vi "Configure Amplitude Sweep at Constant Frequency.vi"(0 "template configuration":refnum<class "SV Signal.lvclass">, 1 "frequency (Hz)":dbl=1000.0, 5 "amplitude range":cluster{"start":dbl, "stop":dbl}={"start"=10.0, "stop"=10000.0} {"stop" format="%.2f"; "start" format="%.2f"}, 7 "number of steps":i32=100 min=1, 9 "profile":enum16{"Linear", "Logarithmic"}(ring)=enum."Logarithmic", 11 "error in (no error)":errorcluster) -> (4 "signal configuration":refnum<class "SV Discrete Sweep.lvclass">, 15 "error out":errorcluster)   [LabVIEW 2017, in "SV Discrete Sweep.lvclass"]
doc: "Configures a user-defined test signal. Wire the outputs to SV Signal (waveform) VI to generate the test signal, or wire to SV Signal Property Node to configure additional parameters before wiring to the SV Signal (waveform) VI."
uses:
  <vilib>/addons/_NISVFA/_Generation/Signal Generation/SV Discrete Sweep/SV Discrete Sweep.lvclass
  C:/Program Files (x86)/National Instruments/LabVIEW 2017/vi.lib/addons/_NISVFA/_Generation/Signal Generation/SV Signal/SV Signal.lvclass
  C:/Program Files (x86)/National Instruments/LabVIEW 2017/vi.lib/addons/_NISVFA/_Generation/Signal Generation/SV Function/SV Function.lvclass
  <vilib>/addons/_NISVFA/_Generation/Signal Generation/SV Signal/SV Signal.lvclass
  <vilib>/addons/_NISVFA/_Generation/Signal Generation/SV Signal/sv_System Timing Model.ctl
  <vilib>/addons/_NISVFA/_Generation/Signal Generation/SV Discrete Sweep/SV Discrete Sweep.lvclass/SV Discrete Sweep.ctl
  <vilib>/addons/_NISVFA/_Generation/Signal Generation/SV Signal/Write Sample Rate.vi
  <vilib>/addons/_NISVFA/_Generation/Signal Generation/SV Signal/Write System Timing Model.vi
  <vilib>/addons/_NISVFA/_Generation/Signal Generation/SV Function/Write Measurement Cycles.vi
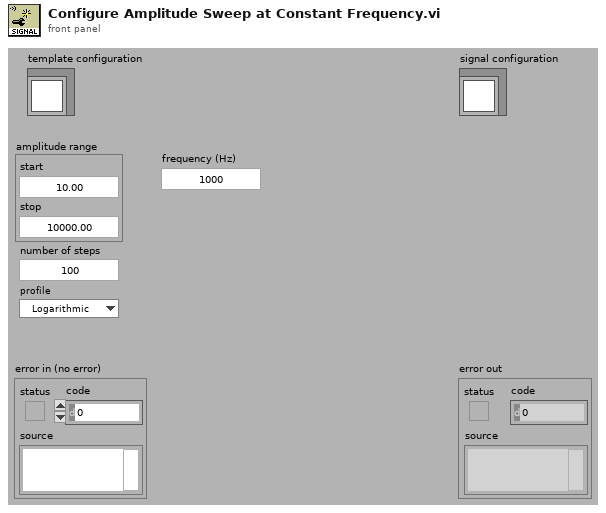
[diagram p1: front panel]
types:
  T1 = cluster{"start":dbl, "stop":dbl, "number of steps":i32}
  T2 = typedef "SV Signal.lvclass/sv_System Timing Model.ctl" = i64
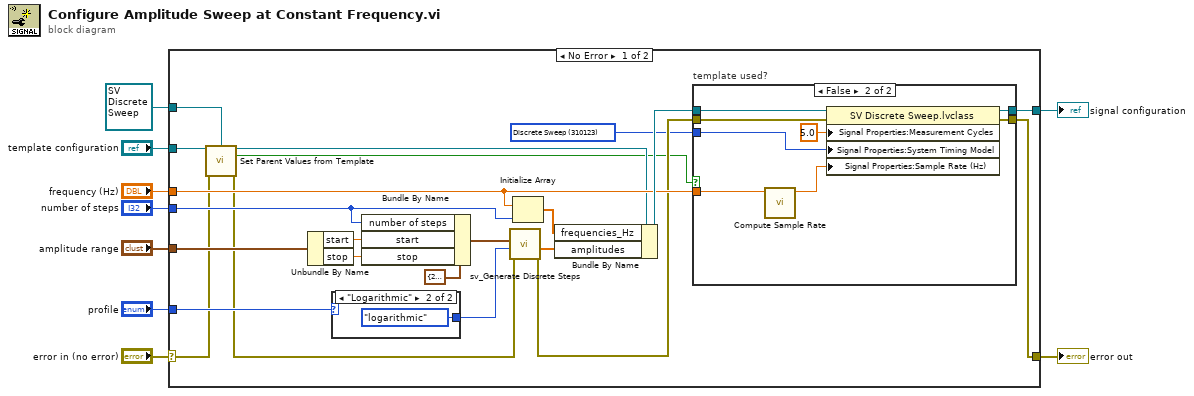
[diagram p0: block diagram]
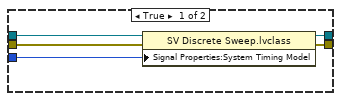
[diagram p2: hidden frame]
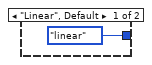
[diagram p3: hidden frame]
diagram:
  n1 = case shown="No Error" "error in (no error)" {
    selector: "error in (no error)" -> [w13 w47]
    tunnel: [w20 w47] -> w8
    tunnel: [w22 w48] -> w6
    tunnel: refnum<class "SV Discrete Sweep.lvclass"> refnum ("Discrete Frequency Sweep") -> [w14 w48]
    tunnel: "amplitude range" -> [w31 _]
    tunnel: "number of steps" -> [w18 _]
    tunnel: "profile" -> [w26 _]
    tunnel: "frequency (Hz)" -> [w19 _]
    tunnel: "template configuration" -> [w16 _]
    frame No Error {
      w10 = T2 310123 items=["Finite"=10178, "-"=-1, "Continuous"=10123, "-"=-2, "Settled"=110123, "Averaged"=210123, "Discrete Sweep"=310123, "Continuous Sweep"=410123] ("System Timing Model")
      n2 = call-dynamic "Set Parent Values from Template.vi"("template configuration"=w16, "signal configuration in"=w14, "error in (no error)"=w13) -> ("signal configuration out"=w15:refnum<class "SV Discrete Sweep.lvclass">, "template used?"=w11:bool, "error out"=w12:errorcluster)  [unwired: 10 in]
      n3 = Unbundle By Name(w31) -> ("start"=w29:dbl, "stop"=w28:dbl)
      n4 = case shown="\"Logarithmic\"" w26 {
        tunnel: [enum16{"linear", "logarithmic"}."linear" ("frequency spacing") enum16{"linear", "logarithmic"}."logarithmic" ("frequency spacing")] -> w25
        frame "Linear", Default {
        }
        frame "Logarithmic" {
        }
      }
      n5 = Bundle By Name(cluster=T1 {"start"=20.0, "stop"=20000.0, "number of steps"=100} ("sweep frequencies"), "number of steps"=w18, "start"=w29, "stop"=w28) -> (w27:T1)
      n6 = call <vilib>:"sv_Generate Discrete Steps.vi"("error in (no error)"=w12, "spacing"=w25, "steps"=w27) -> ("error out"=w17:errorcluster, "frequency list"=w24:dbl[])  [unwired: 7 in]
      n7 = Initialize Array(w19, w18) -> (w21:dbl[])
      n8 = Bundle By Name(cluster=w15, "frequencies_Hz"=w21, "amplitudes"=w24) -> (w23:refnum<class "SV Discrete Sweep.lvclass">)
      n9 = case "template used?" shown="False" w11 {
        tunnel: w23 -> [w36 w44]
        tunnel: [w35 w43] -> w22
        tunnel: [w34 w41] -> w20
        tunnel: w19 -> [_ w40]
        tunnel: w17 -> [w33 w38]
        tunnel: w10 -> [w32 w37]
        frame True {
          n10 = property class="SV Discrete Sweep.lvclass"(reference=w36, error in=w33, "Signal Properties:System Timing Model"=w32) -> (reference out=w35:refnum<class "SV Discrete Sweep.lvclass">, error out=w34:errorcluster)
        }
        frame False {
          n11 = call <vilib>:"Compute Sample Rate.vi"("maximum frequency [Hz]"=w40) -> ("sample rate [Hz]"=w39:dbl)  [unwired: 10 in]
          n12 = property class="SV Discrete Sweep.lvclass"(reference=w44, error in=w38, "Signal Properties:Measurement Cycles"=5.0 ("Measurement Cycles"), "Signal Properties:System Timing Model"=w37, "Signal Properties:Sample Rate (Hz)"=w39) -> (reference out=w43:refnum<class "SV Discrete Sweep.lvclass">, error out=w41:errorcluster)
        }
      }
    }
    frame Error {
    }
  }
  "error out" <- w8
  "signal configuration" <- w6
